vi "Get Variant.vi"(8 "error in (no error)":errorcluster, 11 "Proto Type Common in":refnum<class "Proto Type Data Base.lvclass">) -> (0 "error out":errorcluster, 2 "Value":variant, 3 "Proto Type Common out":refnum<class "Proto Type Data Base.lvclass">)   [LabVIEW 2020, in "Protobuf RAW.lvlib" / "Proto Type Data Base.lvclass"]
uses:
  Proto Type Data Base.lvclass
  Proto Type Data Base.lvclass/Proto Type Data Base.ctl
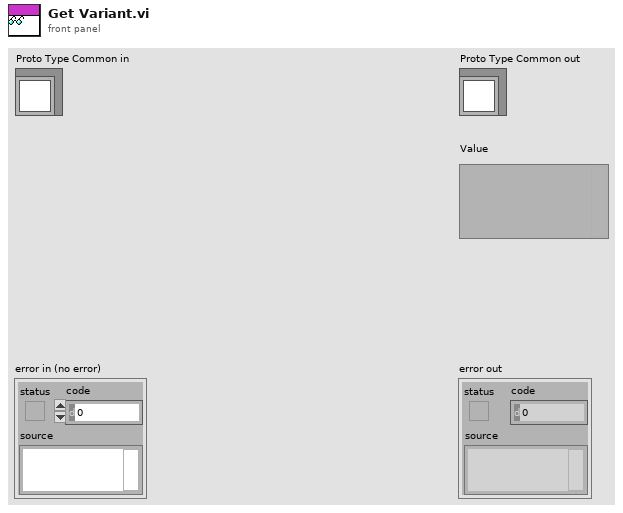
[diagram p1: front panel]
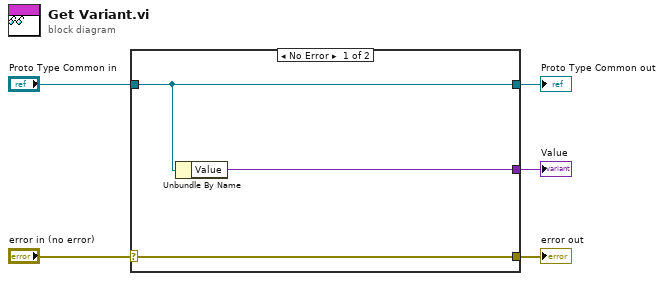
[diagram p0: block diagram]
diagram:
  n1 = case shown="No Error" "error in (no error)" {
    selector: "error in (no error)" -> [w8 w9]
    tunnel: [w8 w9] -> w4
    tunnel: [w7 w10] -> w2
    tunnel: "Proto Type Common in" -> [w7 w10]
    tunnel: [w6 _] -> w1
    frame No Error {
      n2 = Unbundle By Name(w7) -> ("Value"=w6:variant)
    }
    frame Error {
    }
  }
  "error out" <- w4
  "Proto Type Common out" <- w2
  "Value" <- w1
